vi "Write Analogue.vi"(8 "error in (no error)":errorcluster, 9 "Output":bool, 10 "Channel index(0)":i32, 11 "Keysight 5700C in":refnum<class "Keysight 5700C.lvclass">) -> (0 "error out":errorcluster, 2 "Success?":bool, 3 "Keysight 5700C out":refnum<class "Keysight 5700C.lvclass">)   [LabVIEW 2025, in "Power Supply.lvlib" / "Keysight 5700C.lvclass"]
uses:
  Keysight 5700C.lvclass
  Keysight 5700C.lvclass/Keysight 5700C.ctl
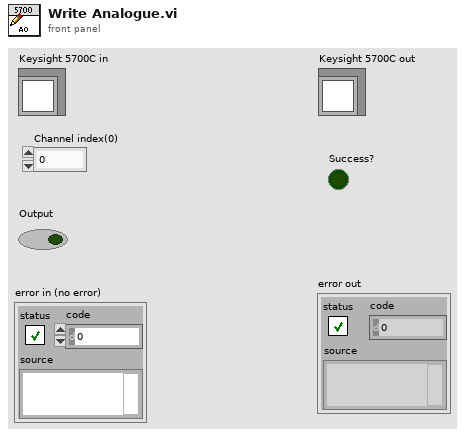
[diagram p1: front panel]
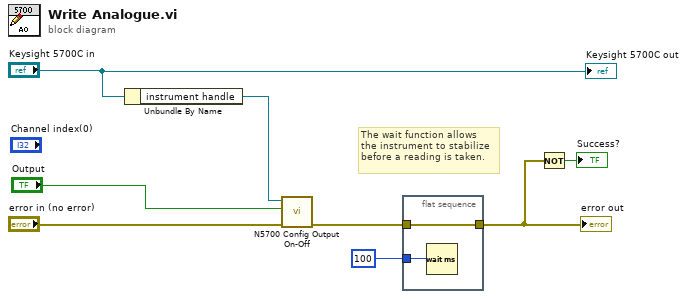
[diagram p0: block diagram]
diagram:
  # "The wait function allows \nthe instrument to stabilize\nbefore a reading is taken."
  n1 = Unbundle By Name("Keysight 5700C in") -> ("instrument handle"=w4:refnum<visa-resource-name>)
  n2 = call <instrlib>:"N5700 Config Output On-Off.vi"("error"="error in (no error)", "Output ON"="Output", "VISA"=w4) -> ("error out"=w2:errorcluster)  [unwired: 4 in, 1 out]
  n3 = flat-sequence {
    tunnel: [w10] -> w1
    tunnel: w2 -> [w10]
    tunnel: u32 100 ("milliseconds to wait") -> [w9]
    frame #0 {
      n4 = Wait (ms)(milliseconds to wait=w9) -> ()  [unwired: 1 out]
    }
  }
  n5 = Not(x=w1) -> (.not. x?=→"Success?":bool)
  "error out" <- w1
  "Keysight 5700C out" <- "Keysight 5700C in"
